vi "Configure TV Trigger Source.vi"(0 "VISA Resource Name":refnum<visa-resource-name>, 1 "Trigger Polarity (Positive)":i32(ring)=1 items=["Negative", "Positive"], 5 "Trigger Source (Channel 1)":string(combo)="CHAN1", 7 "TV Trigger Signal Format (NTSC)":i32(slide), 9 "TV Event (Field 1)":i32(slide), 11 "error in (no error)":errorcluster {"code" format="%.0x"}) -> (4 "VISA Resource Name Out":refnum<visa-resource-name>, 15 "error out":errorcluster {"code" format="%.0x"})   [LabVIEW 2011, in "Agilent 546XX Series.lvlib"]
doc: "This VI configures the TV trigger. You configure the TV trigger source, signal format, the event on which to trigger, and the signal polarity.\n\nNotes:\n\n(1) This VI affects instrument behavior only if the Trigger Type is TV Trigger. Call the ag546xx Configure Trigger VI to set the Trigger Type before you call this VI."
uses:
  Agilent 546XX Series.lvlib
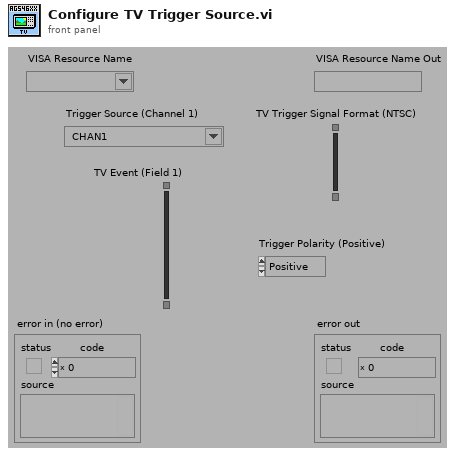
[diagram p1: front panel]
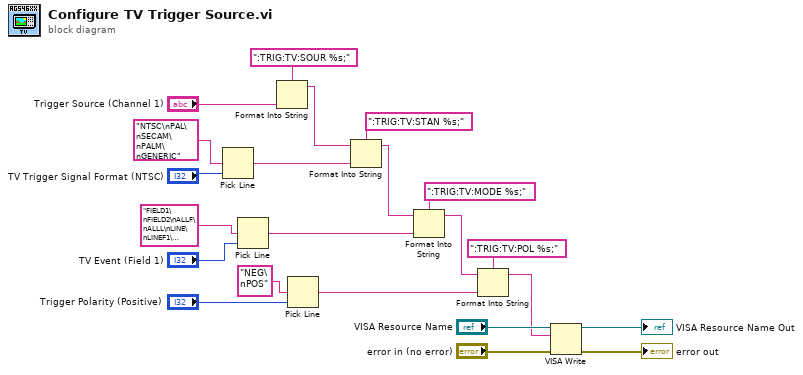
[diagram p0: block diagram]
diagram:
  n1 = Pick Line(multi-line string="NTSC\nPAL\nSECAM\nPALM\nGENERIC", line index="TV Trigger Signal Format (NTSC)") -> (output string=w13:string)  [unwired: 1 in]
  n2 = Pick Line(multi-line string="FIELD1\nFIELD2\nALLF\nALLL\nLINE\nLINEF1\nLINEF2\nLINEA\nLINEV", line index="TV Event (Field 1)") -> (output string=w9:string)  [unwired: 1 in]
  n3 = Format Into String(format string=":TRIG:TV:SOUR %s;", "Trigger Source (Channel 1)") -> (resulting string=w12:string)  [unwired: 2 in, 1 out]
  n4 = Pick Line(multi-line string="NEG\nPOS", line index="Trigger Polarity (Positive)") -> (output string=w3:string)  [unwired: 1 in]
  n5 = Format Into String(format string=":TRIG:TV:STAN %s;", initial string=w12, w13) -> (resulting string=w8:string)  [unwired: 1 in, 1 out]
  n6 = Format Into String(format string=":TRIG:TV:MODE %s;", initial string=w8, w9) -> (resulting string=w6:string)  [unwired: 1 in, 1 out]
  n7 = Format Into String(format string=":TRIG:TV:POL %s;", initial string=w6, w3) -> (resulting string=w1:string)  [unwired: 1 in, 1 out]
  n8 = VISA Write(VISA resource name="VISA Resource Name", write buffer=w1, error in (no error)="error in (no error)") -> (VISA resource name out=→"VISA Resource Name Out":refnum<visa-resource-name>, error out=→"error out":errorcluster)  [unwired: 1 out]
